vi "get available camera registers.vi"() -> (4 "Sorted Device Names":string[](array[string]), 6 "All Registers":T1(array[cluster]), 8 "Camera Registers":T1(array[cluster]), 15 "Found Registers":bool)   [LabVIEW 2010]
uses:
  <vilib>/Utility/file.llb/Read From Spreadsheet File (I64).vi
  <vilib>/Utility/file.llb/Read From Spreadsheet File (string).vi
panel:
  in  "Register":T2
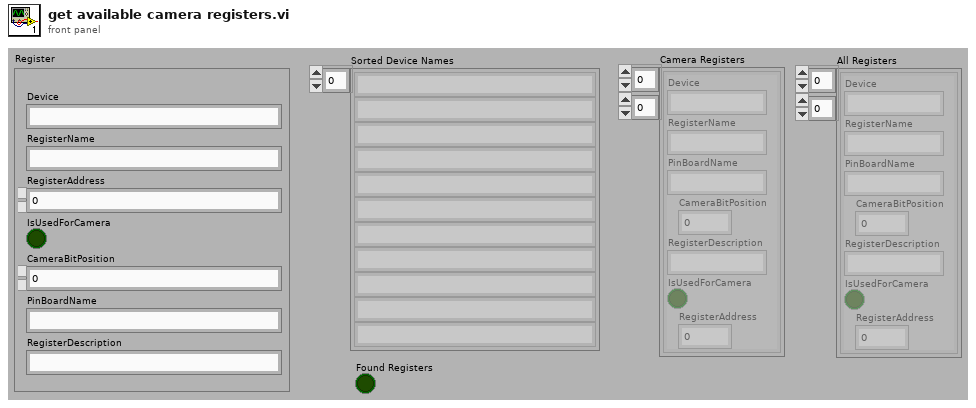
[diagram p1: front panel]
types:
  T1 = cluster{"Device":string, "RegisterName":string, "PinBoardName":string, "CameraBitPosition":i32, "RegisterDescription":string, "IsUsedForCamera":bool, "RegisterAddress":i32}[][]
  T2 = cluster{"Device":string, "RegisterName":string, "PinBoardName":string, "CameraBitPosition":i32, "RegisterDescription":string, "IsUsedForCamera":bool, "RegisterAddress":i32}
  T3 = cluster{"Device":string, "RegisterName":string, "PinBoardName":string, "CameraBitPosition":i32, "RegisterDescription":string, "IsUsedForCamera":bool, "RegisterAddress":i32}[]
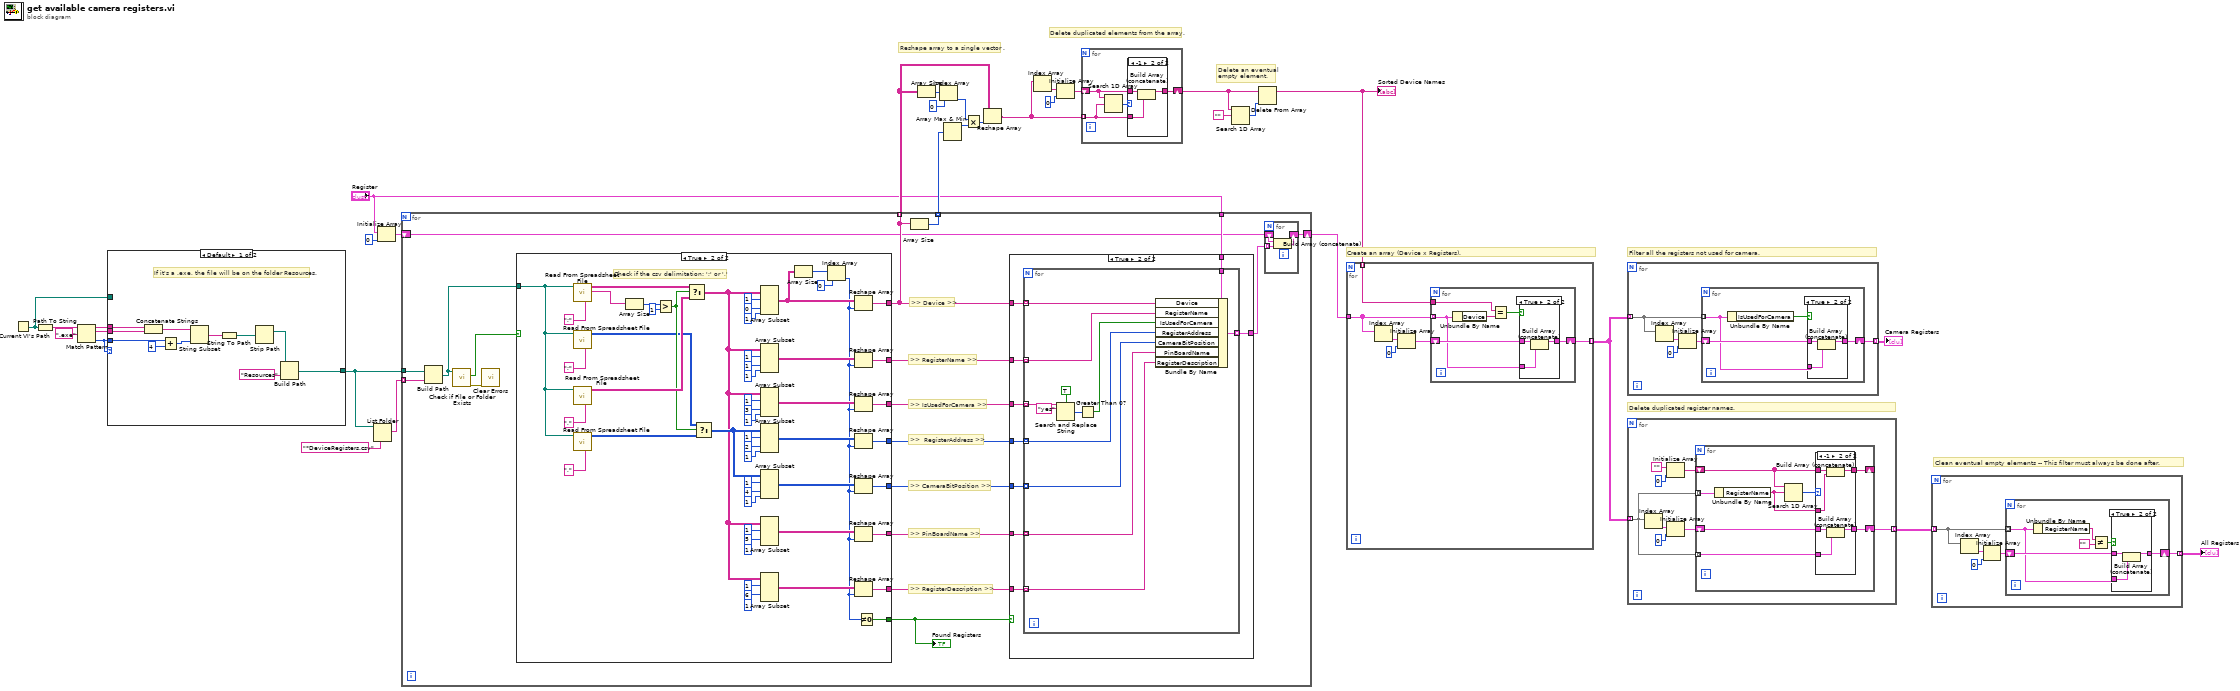
[diagram p0: block diagram]
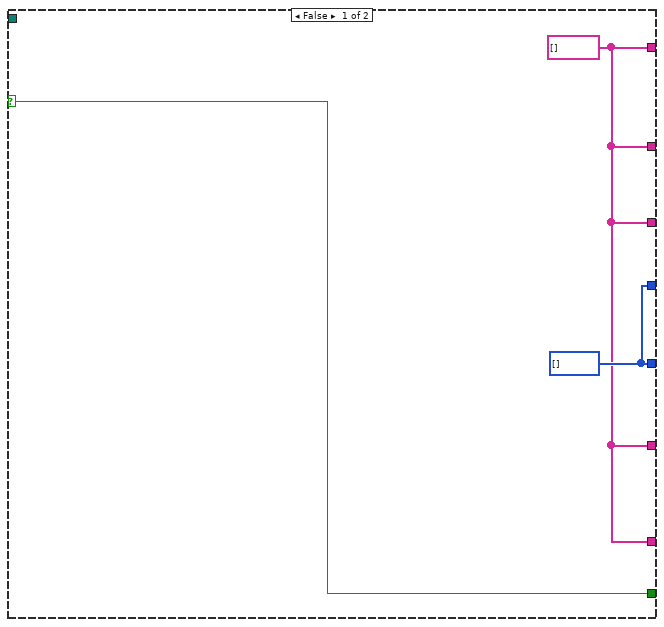
[diagram p8: hidden frame]
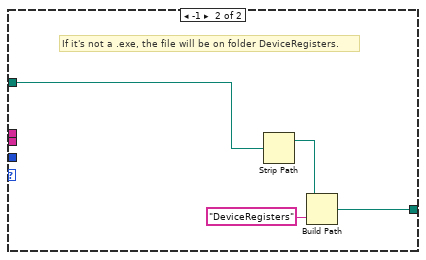
[diagram p9: hidden frame]
diagram:
  # "Clean eventual empty elements -- This filter must always be done after."
  # "Delete duplicated register names."
  # "Filter all the registers not used for camera."
  # "Create an array (Device x Registers)."
  # "Delete an eventual\nempty element."
  # "Delete duplicated elements from the array."
  # "Reshape array to a single vector ."
  n1 = Current VI's Path() -> (path=w27:path)
  n2 = Path To String(path=w27) -> (string=w32:string)
  n3 = Match Pattern(string=w32, regular expression=".exe") -> (before substring=w30:string, match substring=w29:string, offset past match=w28:i32)  [unwired: 1 in, 1 out]
  n4 = case shown="Default" w28 {
    tunnel: [w41 w44] -> w25
    tunnel: w30 -> [w40 _]
    tunnel: w29 -> [w39 _]
    tunnel: w28 -> [w37 _]
    tunnel: w27 -> [_ w45]
    frame Default {
      # "If it's a .exe, the file will be on the folder Resources."
      n5 = Concatenate Strings(w40, w39) -> (w38:string)
      n6 = Add(x=w37, y=4) -> (x+y=w36:i32)
      n7 = String Subset(string=w38, length (rest)=w36) -> (substring=w34:string)  [unwired: 1 in]
      n8 = String To Path(string=w34) -> (path=w33:path)
      n9 = Strip Path(path=w33) -> (stripped path=w43:path)  [unwired: 1 out]
      n10 = Build Path(base path=w43, name or relative path="Resources") -> (appended path=w41:path)
    }
    frame -1 {
      # "If it's not a .exe, the file will be on folder DeviceRegisters."
      n11 = Strip Path(path=w45) -> (stripped path=w47:path)  [unwired: 1 out]
      n12 = Build Path(base path=w47, name or relative path="DeviceRegisters") -> (appended path=w44:path)
    }
  }
  n13 = List Folder(path=w25, pattern="*DeviceRegisters.csv") -> (filenames=w24:string[])  [unwired: 2 in, 3 out]
  n14 = Initialize Array("Register", 0 ("dimension size")) -> (w7:T3)
  n15 = for {
    tunnel: w25 -> [w63]
    tunnel: w24 -> [w61] mode=indexing
    tunnel: [w53] -> w22 mode=indexing
    tunnel: [w52] -> w23 mode=indexing
    shift-right: [w50] -> w5
    shift-left: w7 -> [w49]
    tunnel: "Register" -> [w51]
    # ">> Device >>"
    # ">> RegisterName >>"
    # ">> IsUsedForCamera >>"
    # ">>  RegisterAddress >>"
    # ">> CameraBitPosition >>"
    # ">> RegisterDescription >>"
    # ">> PinBoardName >>"
    n16 = Build Path(base path=w63, name or relative path=w61) -> (appended path=w62:path)
    n17 = call <vilib>:"Check if File or Folder Exists.vi"("path"=w62) -> ("error out"=w65:errorcluster, "file or folder exists?"=w64:bool)  [unwired: 8 in, 1 out]
    n18 = call <vilib>:"Clear Errors.vi"("error in (no error)"=w65) -> ()  [unwired: 6 in, 1 out]
    n19 = case shown="True" w64 {
      selector: w64 -> [w93 _]
      tunnel: w62 -> [_ w141]
      tunnel: [w91 w119] -> w53
      tunnel: [w92 w116] -> w57
      tunnel: [w92 w115] -> w58
      tunnel: [w93 w114] -> w54
      tunnel: [w91 w113] -> w55
      tunnel: [w91 w104] -> w56
      tunnel: [w91 w103] -> w59
      tunnel: [w91 w96] -> w60
      frame False {
        w92 = i64[] []
        w91 = string[] []
      }
      frame True {
        (unwired) 1 ("length")
        (unwired) 1 ("length")
        # "Check if the csv delimitation: ';' or ','"
        n20 = call-poly <vilib>:"Read From Spreadsheet File.vi"("delimiter (\\t)"=";" ("delimiter (\\t)"), "file path (dialog if empty)"=w141) -> ("first row"=w138:string[], "all rows"=w137:string[][])  [unwired: 5 in, 3 out]
        n21 = call-poly <vilib>:"Read From Spreadsheet File.vi"("delimiter (\\t)"=";" ("delimiter (\\t)"), "file path (dialog if empty)"=w141) -> ("all rows"=w134:i64[][])  [unwired: 5 in, 4 out]
        n22 = call-poly <vilib>:"Read From Spreadsheet File.vi"("delimiter (\\t)"="," ("delimiter (\\t)"), "file path (dialog if empty)"=w141) -> ("all rows"=w136:string[][])  [unwired: 5 in, 4 out]
        n23 = call-poly <vilib>:"Read From Spreadsheet File.vi"("delimiter (\\t)"="," ("delimiter (\\t)"), "file path (dialog if empty)"=w141) -> ("all rows"=w133:i64[][])  [unwired: 5 in, 4 out]
        n24 = Array Size(array=w138) -> (size(s)=w140:i32)
        n25 = Greater?(x=w140, y=1) -> (0:w135:bool)
        n26 = Select(t=w137, s=w135, f=w136) -> (s? t:f=w95:string[][])
        n27 = Select(t=w134, s=w135, f=w133) -> (s? t:f=w123:i64[][])
        n28 = Array Subset(array=w95, index (row)=1 ("index"), index (col)=0 ("index"), length (col)=1 ("length")) -> (w120:string[][])  [unwired: 1 in]
        n29 = Array Subset(array=w95, index (row)=1 ("index"), index (col)=1 ("index"), length (col)=1 ("length")) -> (w112:string[][])  [unwired: 1 in]
        n30 = Array Subset(array=w95, index (row)=1 ("index"), index (col)=3 ("index"), length (col)=1 ("length")) -> (w105:string[][])  [unwired: 1 in]
        n31 = Array Subset(array=w123, index (row)=1 ("index"), index (col)=2 ("index"), length (col)=1 ("length")) -> (w118:i64[][])  [unwired: 1 in]
        n32 = Array Subset(array=w123, index (row)=1 ("index"), index (col)=4 ("index"), length (col)=1 ("length")) -> (w117:i64[][])  [unwired: 1 in]
        n33 = Array Subset(array=w95, index (row)=1 ("index"), index (col)=5 ("index")) -> (w102:string[][])  [unwired: 2 in]
        n34 = Array Subset(array=w95, index (row)=1 ("index"), index (col)=6 ("index")) -> (w97:string[][])  [unwired: 2 in]
        n35 = Array Size(array=w120) -> (size(s)=w122:i32[])
        n36 = Index Array(array=w122, index=0) -> (element=w94:i32)
        n37 = Reshape Array(w120, w94) -> (w119:string[])
        n38 = Reshape Array(w112, w94) -> (w113:string[])
        n39 = Reshape Array(w105, w94) -> (w104:string[])
        n40 = Reshape Array(w118, w94) -> (w116:i64[])
        n41 = Reshape Array(w117, w94) -> (w115:i64[])
        n42 = Reshape Array(w102, w94) -> (w103:string[])
        n43 = Reshape Array(w97, w94) -> (w96:string[])
        n44 = Not Equal To 0?(x=w94) -> (x != 0?=w114:bool)
      }
    }
    "Found Registers" <- w54
    n45 = Array Size(array=w53) -> (size(s)=w52:i32)
    n46 = case shown="True" w54 {
      tunnel: w60 -> [_ w77]
      tunnel: w59 -> [_ w76]
      tunnel: w58 -> [_ w75]
      tunnel: w57 -> [_ w74]
      tunnel: w56 -> [_ w73]
      tunnel: w55 -> [_ w72]
      tunnel: w53 -> [_ w71]
      tunnel: [_ w70] -> w48
      tunnel: w51 -> [_ w69]
      frame False {
      }
      frame True {
        n47 = for {
          tunnel: w77 -> [w80] mode=indexing
          tunnel: w76 -> [w81] mode=indexing
          tunnel: w75 -> [w82] mode=indexing
          tunnel: w74 -> [w83] mode=indexing
          tunnel: w73 -> [w90] mode=indexing
          tunnel: w72 -> [w85] mode=indexing
          tunnel: w71 -> [w84] mode=indexing
          tunnel: [w79] -> w70 mode=indexing
          tunnel: w69 -> [w78]
          n48 = Search and Replace String(case sensitive?=TRUE ("ignore case? (F)"), input string=w90, search string="yes") -> (number of replacements=w87:i32)  [unwired: 5 in, 3 out]
          n49 = Greater Than 0?(x=w87) -> (x > 0?=w86:bool)
          n50 = Bundle By Name(cluster=w78, "Device"=w84, "RegisterName"=w85, "IsUsedForCamera"=w86, "RegisterAddress"=w83, "CameraBitPosition"=w82, "PinBoardName"=w81, "RegisterDescription"=w80) -> (w79:T2)
        }
      }
    }
    n51 = for {
      tunnel: w48 -> [w66] mode=indexing
      shift-right: [w68] -> w50
      shift-left: w49 -> [w67]
      n52 = Build Array (concatenate)(w67, w66) -> (w68:T3)
    }
  }
  n53 = Array Size(array=w22) -> (size(s)=w20:i32[])
  n54 = Index Array(array=w20, index=0) -> (element=w17:i32)
  n55 = Array Max & Min(array=w23) -> (max value=w18:i32)  [unwired: 3 out]
  n56 = Multiply(x=w17, y=w18) -> (x*y=w19:i32)
  n57 = Reshape Array(w22, w19) -> (w13:string[])
  n58 = Index Array(array=w13) -> (element=w14:string)  [unwired: 1 in]
  n59 = Initialize Array(w14, 0 ("Dimension Size")) -> (w15:string[])
  n60 = for {
    tunnel: w13 -> [w148] mode=indexing
    shift-right: [w147] -> w11
    shift-left: w15 -> [w146]
    n61 = Search 1D Array(1D array=w146, element=w148) -> (index of element=w149:i32)  [unwired: 1 in]
    n62 = case shown="-1" w149 {
      tunnel: w148 -> [_ w153]
      tunnel: [w150 w151] -> w147
      tunnel: w146 -> [w150 w152]
      frame Default {
      }
      frame -1 {
        n63 = Build Array (concatenate)(w152, w153) -> (w151:string[])
      }
    }
  }
  n64 = Search 1D Array(1D array=w11, element="") -> (index of element=w10:i32)  [unwired: 1 in]
  n65 = Delete From Array(array=w11, index=w10) -> (array with subset deleted=w9:string[])  [unwired: 1 in, 1 out]
  "Sorted Device Names" <- w9
  n66 = for {
    tunnel: w9 -> [w159] mode=indexing
    tunnel: w5 -> [w156]
    tunnel: [w154] -> w4 mode=indexing
    n67 = Index Array(array=w156) -> (element=w158:T2)  [unwired: 1 in]
    n68 = Initialize Array(w158, 0 ("Dimension Size")) -> (w155:T3)
    n69 = for {
      tunnel: w159 -> [w162]
      tunnel: w156 -> [w160] mode=indexing
      shift-right: [w164] -> w154
      shift-left: w155 -> [w165]
      n70 = Unbundle By Name(w160) -> ("Device"=w163:string)
      n71 = Equal?(x=w162, y=w163) -> (x = y?=w161:bool)
      n72 = case shown="True" w161 {
        tunnel: [w166 w168] -> w164
        tunnel: w165 -> [w166 w169]
        tunnel: w160 -> [_ w167]
        frame False {
        }
        frame True {
          n73 = Build Array (concatenate)(w169, w167) -> (w168:T3)
        }
      }
    }
  }
  n74 = for {
    tunnel: w4 -> [w172] mode=indexing
    tunnel: [w170] -> w2 mode=indexing
    n75 = Index Array(array=w172) -> (element=w174:T2)  [unwired: 1 in]
    n76 = Initialize Array(w174, 0 ("Dimension Size")) -> (w171:T3)
    n77 = for {
      tunnel: w172 -> [w176] mode=indexing
      shift-right: [w177] -> w170
      shift-left: w171 -> [w178]
      n78 = Unbundle By Name(w176) -> ("IsUsedForCamera"=w175:bool)
      n79 = case shown="True" w175 {
        tunnel: [w179 w181] -> w177
        tunnel: w178 -> [w179 w182]
        tunnel: w176 -> [_ w180]
        frame False {
        }
        frame True {
          n80 = Build Array (concatenate)(w182, w180) -> (w181:T3)
        }
      }
    }
  }
  "Camera Registers" <- w2
  n81 = for {
    tunnel: w4 -> [w184] mode=indexing
    tunnel: [w183] -> w3 mode=indexing
    n82 = Index Array(array=w184) -> (element=w190:T2)  [unwired: 1 in]
    n83 = Initialize Array("", 0 ("Dimension Size")) -> (w185:string[])
    n84 = Initialize Array(w190, 0 ("Dimension Size")) -> (w189:T3)
    n85 = for {
      tunnel: w184 -> [w198] mode=indexing
      shift-right: [w197] -> w183
      shift-left: w189 -> [w196]
      shift-right: [w195] -> _
      shift-left: w185 -> [w194]
      tunnel: w184 -> [w193] mode=indexing
      n86 = Unbundle By Name(w193) -> ("RegisterName"=w191:string)
      n87 = Search 1D Array(1D array=w194, element=w191) -> (index of element=w192:i32)  [unwired: 1 in]
      n88 = case shown="-1" w192 {
        tunnel: w198 -> [_ w206]
        tunnel: [w200 w204] -> w197
        tunnel: w196 -> [w200 w205]
        tunnel: [w199 w202] -> w195
        tunnel: w194 -> [w199 w203]
        tunnel: w191 -> [_ w201]
        frame Default {
        }
        frame -1 {
          n89 = Build Array (concatenate)(w203, w201) -> (w202:string[])
          n90 = Build Array (concatenate)(w205, w206) -> (w204:T3)
        }
      }
    }
  }
  n91 = for {
    tunnel: w3 -> [w209] mode=indexing
    tunnel: [w207] -> w1 mode=indexing
    n92 = Index Array(array=w209) -> (element=w211:T2)  [unwired: 1 in]
    n93 = Initialize Array(w211, 0 ("Dimension Size")) -> (w208:T3)
    n94 = for {
      tunnel: w209 -> [w215] mode=indexing
      shift-right: [w216] -> w207
      shift-left: w208 -> [w217]
      n95 = Unbundle By Name(w215) -> ("RegisterName"=w213:string)
      n96 = Not Equal?(x=w213, y="") -> (x != y?=w212:bool)
      n97 = case shown="True" w212 {
        tunnel: [w218 w220] -> w216
        tunnel: w217 -> [w218 w221]
        tunnel: w215 -> [_ w219]
        frame False {
        }
        frame True {
          n98 = Build Array (concatenate)(w221, w219) -> (w220:T3)
        }
      }
    }
  }
  "All Registers" <- w1
